vi "CRC-U8.vi"(5 "Polynom":u8=213 format="%02x", 7 "Start":u8=255 format="%02x", 11 "Send":u8[](array[numeric])=[9, 1, 2, 64, 96, 0, 6, 0] format="%02x") -> (3 "CRC":u8=44 format="%x")   [LabVIEW 2011]
panel:
  # "53,9,1,2,40,60,00,06,00,2C,45"
  # "hier muss 2C rauskommen"
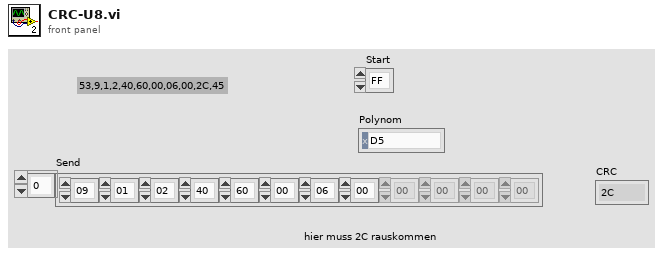
[diagram p1: front panel]
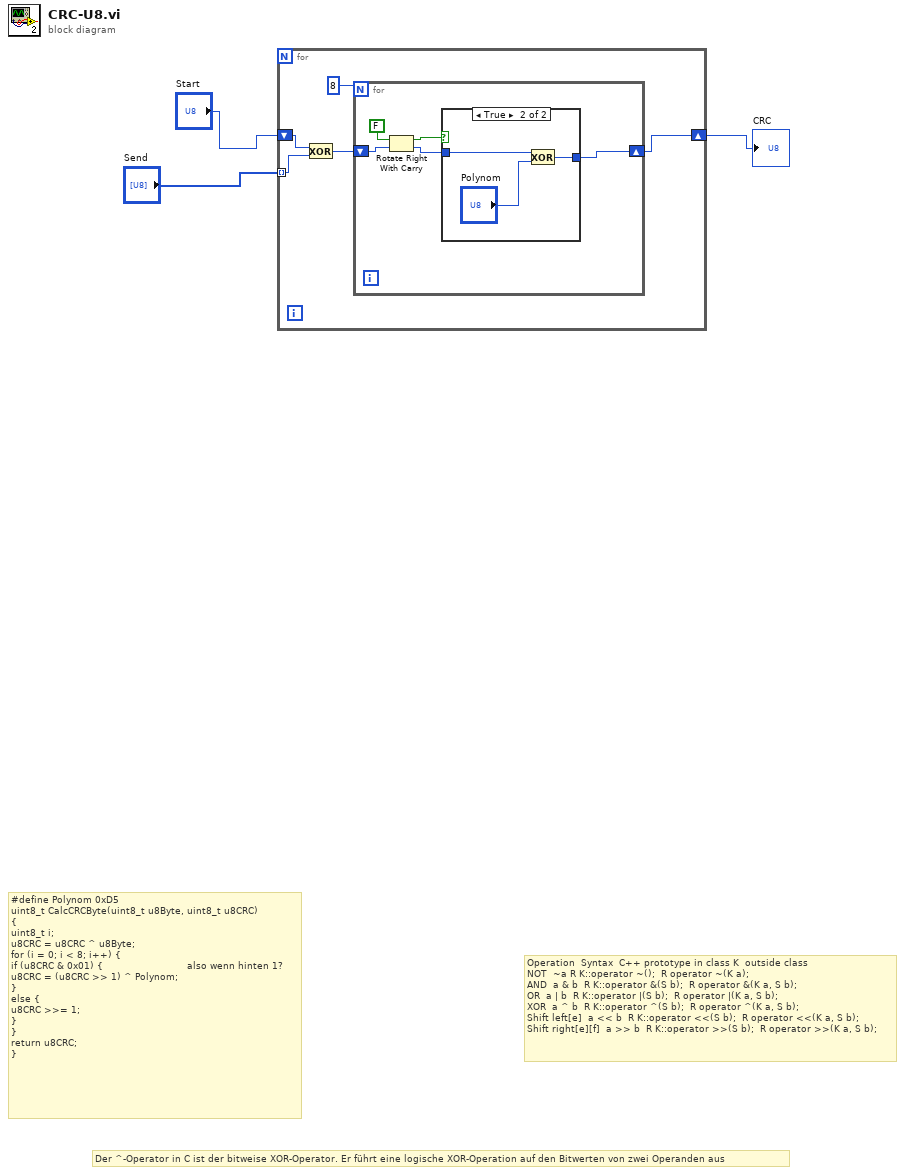
[diagram p0: block diagram]
diagram:
  # "Operation \tSyntax \tC++ prototype in class K \toutside class\nNOT \t~a\tR K::operator ~(); \tR operator ~(K a);\nAND \ta & b \tR K::operator &(S b); \tR operator &(K a, S b);\nOR \ta | b \tR K::operator |(S b); \tR operator |(K a, S b);\nXOR \ta ^ b \tR K::operator ^(S b); \tR operator ^(K a, S b);\nShift left[e] \ta << b \tR K::operator <<(S b); \tR operator <<(K a, S b);\nShift right[e][f] \ta >> b \tR K::operator >>(S b); \tR operator >>(K a, S b);"
  # "#define Polynom 0xD5\nuint8_t CalcCRCByte(uint8_t u8Byte, uint8_t u8CRC)\n{\nuint8_t i;\nu8CRC = u8CRC ^ u8Byte;\nfor (i = 0; i < 8; i++) {\nif (u8CRC & 0x01) {                            also wenn hinten 1?\nu8CRC = (u8CRC >> 1) ^ Polynom;\n}\nelse {\nu8CRC >>= 1;\n}\n}\nreturn u8CRC;\n}"
  # "Der ^-Operator in C ist der bitweise XOR-Operator. Er führt eine logische XOR-Operation auf den Bitwerten von zwei Operanden aus"
  n1 = for {
    tunnel: "Send" -> [w7] mode=indexing
    shift-right: [w5] -> w1
    shift-left: "Start" -> [w8]
    n2 = Exclusive Or(1:w7, 2:w8) -> (0:w6:u8)
    n3 = for {
      N: 8 -> [_]
      shift-right: [w9] -> w5
      shift-left: w6 -> [w12]
      n4 = Rotate Right With Carry(2:w12, 3:FALSE ("carry")) -> (0:w10:u8, 1:w11:bool)
      n5 = case shown="True" w11 {
        tunnel: [w14 w16] -> w9
        tunnel: w10 -> [w14 w15]
        frame False {
        }
        frame True {
          n6 = Exclusive Or(1:"Polynom", 2:w15) -> (0:w16:u8)
        }
      }
    }
  }
  "CRC" <- w1
